vi "GlobalScanningPositionInPixelValues.vi"() -> ()   [LabVIEW 2011]
panel:
  in  "Pos Pixel Z":dbl
  in  "Pos Pixel Y":dbl
  in  "Pos Pixel X":dbl
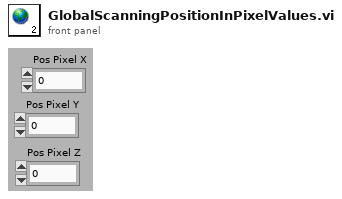
[diagram p1: front panel]
diagram:
